vi "Renishaw-XL80_GetMatTemp.vi"(8 "error in (no error)":errorcluster, 11 "Renishaw-XL80 in":refnum<class "Renishaw-XL80.lvclass">) -> (0 "error out":errorcluster, 1 "pStatus Array":i32[](array[ring]) items=["SENSOR_OK"=0, "SENSOR_BAD_READING"=1, "SENSOR_FAILED"=2, "SENSOR_NOT_CONNECTED"=4], 2 "Temperature Array":dbl[](array[numeric]), 3 "Renishaw-XL80 out":refnum<class "Renishaw-XL80.lvclass">)   [LabVIEW 2024, in "Renishaw-XL80.lvclass"]
doc: "This method disconnects a client from a DX10.\n\nDefinition\nHRESULTGetMatTemp( [in] short nIndex, [out] SENSOR_STATUS_CODES *pStatus, [out, retval] double *pVal);\nParameters\nnIndex\nIdentifies the sensor to be read from. Its value should be in [1..3].\n\npStatus\nA variable that will be set to one of the SENSOR_STATUS_CODES.\n\npVal\nA variable that will be set to the material temperature reading from the specified sensor (in oC).\n\nComments\nThis method will return with an HRESULT of E_INVALIDARG if nIndex is not in [1..3].\n\nIf the client has not connected to the DX10 then the default value (20oC) will be returned and the status will be set to SENSOR_NOT_CONNECTED.\n\nIf the client connected to a DX10 and it subsequently stopped responding, or the EC10 stopped responding then the last values obtained from the EC10 will be returned i.e. the status will not be modified. It is important therefore to monitor both the DX10Status and EC10Status. This is easily done using the _RenishawDX10Events interface.\n\n\nIf the sensor status is SENSOR_NOT_CONNECTED or SENSOR_BAD_READING, then pVal will be set to the last known valid reading.\n\nThe property will normally return an HRESULT of S_OK. However, it will return E_POINTER if the client supplies a null pointer for either pVal or pStatus."
uses:
  Renishaw-XL80.lvclass
  Renishaw-XL80.lvclass/Renishaw-XL80.ctl
  D:/A.C.M/Example CSharp_64/bin/Debug/Interop.DX10SDKADAPTORLib.dll
  A.C.M/Example CSharp_64/bin/Debug/Interop.DX10SDKADAPTORLib.dll
panel:
  out "pStatus":i32(ring) items=["SENSOR_OK"=0, "SENSOR_BAD_READING"=1, "SENSOR_FAILED"=2, "SENSOR_NOT_CONNECTED"=4]
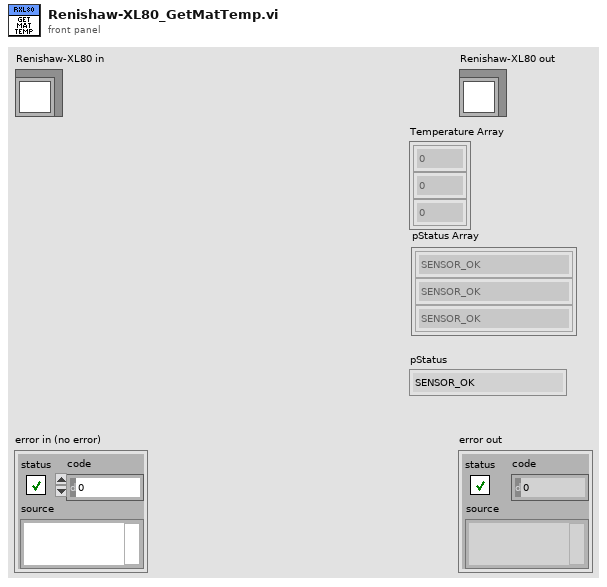
[diagram p1: front panel]
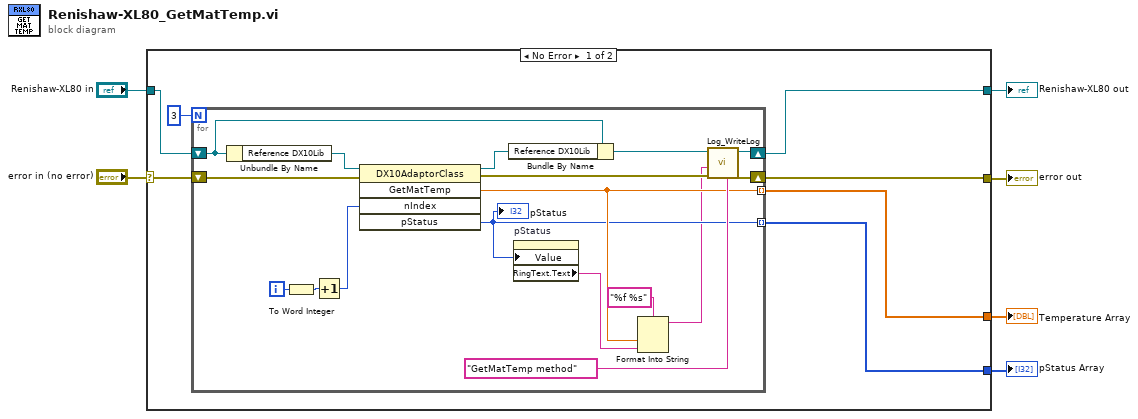
[diagram p0: block diagram]
diagram:
  n1 = case shown="No Error" "error in (no error)" {
    selector: "error in (no error)" -> [w13 w32]
    tunnel: [w9 w32] -> w5
    tunnel: [w10 w31] -> w3
    tunnel: "Renishaw-XL80 in" -> [w11 w31]
    tunnel: [w8 _] -> w2
    tunnel: [w7 _] -> w1
    frame No Error {
      n2 = for {
        N: 3 -> [_]
        shift-right: [w21] -> w10
        shift-left: w11 -> [w23]
        shift-right: [w24] -> w9
        shift-left: w13 -> [w30]
        tunnel: [w18] -> w8 mode=indexing
        tunnel: [w17] -> w7 mode=indexing
        i -> [w28]
        n3 = Unbundle By Name(w23) -> ("Reference DX10Lib"=w26:refnum<k24>)
        n4 = To Word Integer(number=w28) -> (16bit integer=w27:i16)
        n5 = Increment(x=w27) -> (x+1=w29:i16)
        n6 = invoke class="DX10AdaptorClass" method="GetMatTemp"(reference=w26, error in=w30, "nIndex"=w29) -> (reference out=w25:refnum<k24>, error out=w15:errorcluster, "GetMatTemp"=w18:dbl, "pStatus"=w17:i32)  [unwired: 2 in, 1 out]
        "pStatus" <- w17
        n7 = Bundle By Name(cluster=w23, "Reference DX10Lib"=w25) -> (w22:refnum<class "Renishaw-XL80.lvclass">)
        n8 = property on="pStatus" class="Ring (strict)"("Value"=w17) -> ("RingText.Text"=w16:string)  [unwired: 2 in, 2 out]
        n9 = Format Into String(format string="%f %s", w18, w16) -> (resulting string=w14:string)  [unwired: 2 in, 1 out]
        n10 = call-dynamic "Log_WriteLog.vi"("Additional text"="GetMatTemp method", "error in (no error)"=w15, "Response"=w14, "Log in"=w22) -> ("error out"=w24:errorcluster, "Log out"=w21:refnum<class "Renishaw-XL80.lvclass">)  [unwired: 6 in]
      }
    }
    frame Error {
    }
  }
  "error out" <- w5
  "Renishaw-XL80 out" <- w3
  "Temperature Array" <- w2
  "pStatus Array" <- w1
